vi "StartDBControlVI.vi"(8 "entrée d'erreur (pas d'erreur)":errorcluster, 11 "Control en entrée":refnum<class "Control-Server.lvclass">) -> (0 "sortie d'erreur":errorcluster, 3 "Control en sortie":refnum<class "Control-Server.lvclass">)   [LabVIEW 2020, in "Control-Server.lvclass"]
uses:
  Classes/Control/Control-Server/Control-Server.lvclass
  C:/dev/TRANCON/Classes/GeneralFunctionality/GeneralFunctionality.lvclass
  Classes/Control/Control-Server/Control-Server.lvclass/Control-Server.ctl
  Clusters-def/Message types.ctl
  Classes/Message/Message.lvclass/Message.ctl
  Classes/DB/DB.lvclass
  Classes/Message/Message.lvclass
  Classes/GeneralFunctionality/GeneralFunctionality.lvclass
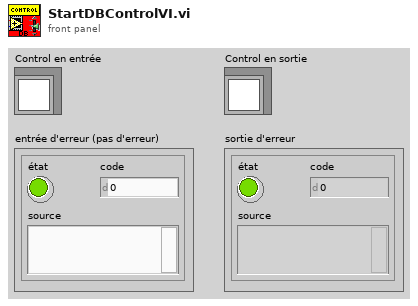
[diagram p1: front panel]
types:
  T1 = typedef "Message types.ctl" = string
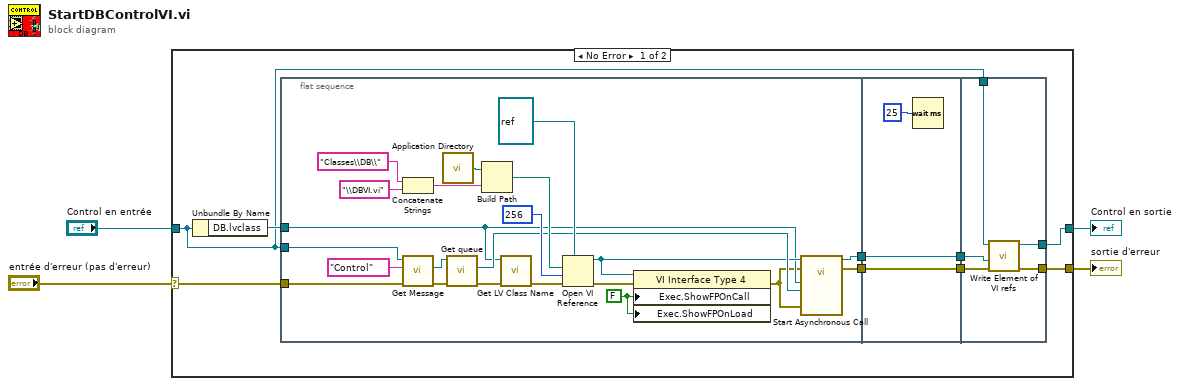
[diagram p0: block diagram]
diagram:
  n1 = case shown="No Error" "entrée d'erreur (pas d'erreur)" {
    selector: "entrée d'erreur (pas d'erreur)" -> [w5 w45]
    tunnel: [w13 w45] -> w4
    tunnel: "Control en entrée" -> [w6 w44]
    tunnel: [w12 w44] -> w2
    frame No Error {
      n2 = Unbundle By Name(w6) -> ("DB.lvclass"=w7:refnum<class "DB.lvclass">)
      n3 = flat-sequence {
        tunnel: [w22] -> w11
        tunnel: w7 -> [w15]
        tunnel: [w21] -> w9
        tunnel: w5 -> [w24]
        tunnel: w6 -> [w25]
        tunnel: w11 -> [w38]
        tunnel: [w38] -> w10
        tunnel: w9 -> [w37]
        tunnel: [w37] -> w8
        tunnel: [w40] -> w13
        tunnel: w10 -> [w39]
        tunnel: w6 -> [w41]
        tunnel: [w43] -> w12
        tunnel: w8 -> [w42]
        frame #0 {
          w29 = FALSE ("Execution:Show Front Panel On Call")
          n4 = Concatenate Strings("Classes\\DB\\" ("chaîne"), "\\DBVI.vi" ("chaîne")) -> (w28:string)
          n5 = call "Get Message.vi"("error in (no error)"=w24, "Message type"=T1 "Control", "GeneralFunctionality en entrée"=w25) -> ("error out"=w19:errorcluster, "Message.lvclass"=w20:refnum<class "Message.lvclass">)  [unwired: 6 in, 1 out]
          n6 = call <vilib>:"Application Directory.vi"() -> ("Application Directory"=w33:path)
          n7 = call "Get queue.vi"("error in (no error)"=w19, "Message in"=w20) -> ("error out"=w16:errorcluster, "queue"=w18:refnum<queue>)  [unwired: 7 in, 1 out]
          n8 = Build Path(base path=w33, name or relative path=w28) -> (appended path=w34:path)
          n9 = call <vilib>:"Get LV Class Name.vi"("error in (no error)"=w16, "object"=w15) -> ("error out"=w35:errorcluster)  [unwired: 8 in, 1 out]
          n10 = Open VI Reference(type specifier VI Refnum (for type only)=refnum<vi> refnum ("spécificateur de type du refnum de VI (pour type seulement)"), vi path=w34, options=256, error in (no error)=w35) -> (vi reference=w17:refnum<vi>, error out=w30:errorcluster)  [unwired: 2 in]
          n11 = property class="VI Interface Type 4"(reference=w17, error in=w30, "Exec.ShowFPOnCall"=w29, "Exec.ShowFPOnLoad"=w29) -> (error out=w14:errorcluster)  [unwired: 1 out]
          n12 = call-by-ref "Start Asynchronous Call"(reference=w17, error in=w14, 8:"error in (no error)"=w14, "ControlQueue"=w18, "DB in"=w15) -> (reference out=w21:refnum<vi>, error out=w22:errorcluster)  [unwired: 8 in, 1 out]
        }
        frame #1 {
          n13 = Wait (ms)(milliseconds to wait=u32 25) -> ()  [unwired: 1 out]
        }
        frame #2 {
          n14 = call "Write Element of VI refs.vi"("error in (no error)"=w39, "vi reference"=w42, "Control in"=w41) -> ("error out"=w40:errorcluster, "Control out"=w43:refnum<class "Control-Server.lvclass">)  [unwired: 7 in]
        }
      }
    }
    frame Error {
    }
  }
  "sortie d'erreur" <- w4
  "Control en sortie" <- w2
